vi "SDO_TRAJECTORY_EXECUTE_ABS.vi"(6 "EnableClosedLoop":bool=TRUE, 8 "Init":bool, 11 "End Pose ENG":T1={"TRANSLATION"={"X"=0.0, "Y"=0.0}, "ROTATION"={"VALUE"=0.0, "COS"=1.0, "SIN"=0.0}} {"ROTATION"."SIN" format="%13.4f"; "ROTATION"."COS" format="%13.4f"; "ROTATION"."VALUE" format="%13.4f"; "TRANSLATION"."Y" format="%14.3f"; "TRANSLATION"."X" format="%14.3f"}) -> (0 "AtReference":bool, 3 "Chassis Velocity Target":T4 {"vOmega" format="%10.3f"; "vY" format="%10.3f"; "vX" format="%10.3f"})   [LabVIEW 2019]
uses:
  <vilib>/Rock Robotics/WPI/ThirdParty/JAS_Junk/TrajLib/TypeDef/CHASSIS_SPEEDS.ctl
  <vilib>/Rock Robotics/WPI/ThirdParty/JAS_Junk/TrajLib/TypeDef/POSE2D.ctl
  <vilib>/Rock Robotics/WPI/ThirdParty/JAS_Junk/TrajLib/TypeDef/TRANSLATION2D.ctl
  <vilib>/Rock Robotics/WPI/ThirdParty/JAS_Junk/TrajLib/TypeDef/ROTATION2D.ctl
  <vilib>/Rock Robotics/WPI/ThirdParty/JAS_Junk/TrajLib/VI/Util_GetTime_U32.vi
  <vilib>/Rock Robotics/WPI/ThirdParty/JAS_Junk/TrajLib/ProfiledPIDController_NewPeriod.vi
  <vilib>/Rock Robotics/WPI/ThirdParty/JAS_Junk/TrajLib/ProfiledPIDController_SetIntegratorRange.vi
  <vilib>/Rock Robotics/WPI/ThirdParty/JAS_Junk/TrajLib/ProfiledPIDController_DisableContInput.vi
  <vilib>/Rock Robotics/WPI/ThirdParty/JAS_Junk/TrajLib/ProfiledPIDController_EnableContInput.vi
  <vilib>/Rock Robotics/WPI/ThirdParty/JAS_Junk/TrajLib/TrapProfConstraint_New.vi
  <vilib>/Rock Robotics/WPI/ThirdParty/JAS_Junk/TrajLib/HolDrvCtrl_New.vi
  <vilib>/Rock Robotics/WPI/ThirdParty/JAS_Junk/TrajLib/HolDrvCtrl_PackPID.vi
  <vilib>/Rock Robotics/WPI/ThirdParty/JAS_Junk/TrajLib/HolDrvCtrl_SetTolerance.vi
  <vilib>/Rock Robotics/WPI/ThirdParty/JAS_Junk/TrajLib/HolDrvCtrl_SetEnabled.vi
  <vilib>/Rock Robotics/WPI/ThirdParty/JAS_Junk/TrajLib/HolDrvCtrl_Calculate_Trajectory.vi
  <vilib>/Rock Robotics/WPI/ThirdParty/JAS_Junk/TrajLib/HolDrvCtrl_AtReference.vi
  <vilib>/Rock Robotics/WPI/ThirdParty/JAS_Junk/TrajLib/TrapProfState_New.vi
  <vilib>/Rock Robotics/WPI/ThirdParty/JAS_Junk/TrajLib/PIDController_NewPeriod.vi
  <vilib>/Rock Robotics/SystemInterfaces/NetworkCommunication/NetComm_UsageReport_report.vi
  <vilib>/Rock Robotics/WPI/ThirdParty/JAS_Junk/TrajLib/PIDController_SetIntegratorRange.vi
  <vilib>/Rock Robotics/WPI/ThirdParty/JAS_Junk/TrajLib/PIDController_DisableContinousInput.vi
  <vilib>/Rock Robotics/WPI/ThirdParty/JAS_Junk/TrajLib/PIDController_EnableContinousInput.vi
  <vilib>/Rock Robotics/WPI/ThirdParty/JAS_Junk/TrajLib/Conv_Deg_Radians.vi
  <vilib>/Rock Robotics/WPI/ThirdParty/JAS_Junk/TrajLib/PIDController_Reset.vi
  <vilib>/Rock Robotics/WPI/ThirdParty/JAS_Junk/TrajLib/HolDrvCtrl_Calculate.vi
  <vilib>/Rock Robotics/WPI/ThirdParty/JAS_Junk/TrajLib/Rotation2d_GetRadians.vi
  <vilib>/Rock Robotics/WPI/ThirdParty/JAS_Junk/TrajLib/Rotation2d_GetAngleCosSin.vi
  <vilib>/Rock Robotics/WPI/ThirdParty/JAS_Junk/TrajLib/Pose2d_RelativeTo.vi
  <vilib>/Rock Robotics/WPI/ThirdParty/JAS_Junk/TrajLib/Pose2d_getRotation.vi
  <vilib>/Rock Robotics/WPI/ThirdParty/JAS_Junk/TrajLib/Rotation2d_Minus.vi
  <vilib>/Rock Robotics/WPI/ThirdParty/JAS_Junk/TrajLib/ProfiledPIDController_Calculate_Meas_Goal.vi
  <vilib>/Rock Robotics/WPI/ThirdParty/JAS_Junk/TrajLib/ChassisSpeeds_FromFieldRelativeSpeeds.vi
  <vilib>/Rock Robotics/WPI/ThirdParty/JAS_Junk/TrajLib/PIDController_Calculate_SP_PV.vi
  <vilib>/Rock Robotics/WPI/ThirdParty/JAS_Junk/TrajLib/ProfiledPIDController_Reset_PosOnly.vi
  <vilib>/Rock Robotics/WPI/ThirdParty/JAS_Junk/TrajLib/Transform2d_Create_PosePose.vi
  <vilib>/Rock Robotics/WPI/ThirdParty/JAS_Junk/TrajLib/Pose2d_New_TRRO.vi
  <vilib>/Rock Robotics/WPI/ThirdParty/JAS_Junk/TrajLib/Rotation2d_UnaryMinus.vi
  <vilib>/Rock Robotics/WPI/ThirdParty/JAS_Junk/TrajLib/Rotation2d_RotateBy.vi
  <vilib>/Rock Robotics/WPI/ThirdParty/JAS_Junk/TrajLib/ProfiledPIDController_SetGoal_PosOnly.vi
  <vilib>/Rock Robotics/WPI/ThirdParty/JAS_Junk/TrajLib/ProfiledPIDController_Calculate_Meas.vi
  <vilib>/Rock Robotics/WPI/ThirdParty/JAS_Junk/TrajLib/Rotation2d_GetCos.vi
  <vilib>/Rock Robotics/WPI/ThirdParty/JAS_Junk/TrajLib/Rotation2d_GetSin.vi
  <vilib>/Rock Robotics/WPI/ThirdParty/JAS_Junk/TrajLib/PIDController_SetSetpoint.vi
  <vilib>/Rock Robotics/WPI/ThirdParty/JAS_Junk/TrajLib/PIDController_Calculate_PV.vi
  <vilib>/Rock Robotics/WPI/ThirdParty/JAS_Junk/TrajLib/ProfiledPIDController_Reset.vi
  <vilib>/Rock Robotics/WPI/ThirdParty/JAS_Junk/TrajLib/Translation2d_RotateBy.vi
  <vilib>/Rock Robotics/WPI/ThirdParty/JAS_Junk/TrajLib/Translation2d_Minus.vi
  <vilib>/Rock Robotics/WPI/ThirdParty/JAS_Junk/TrajLib/Rotation2d_CreateAngle.vi
  <vilib>/Rock Robotics/WPI/ThirdParty/JAS_Junk/TrajLib/Rotation2d_CreateXY.vi
  <vilib>/Rock Robotics/WPI/ThirdParty/JAS_Junk/TrajLib/ProfiledPIDController_SetGoal.vi
  <vilib>/Rock Robotics/WPI/ThirdParty/JAS_Junk/TrajLib/TrapProfile_New.vi
  <vilib>/Rock Robotics/WPI/ThirdParty/JAS_Junk/TrajLib/ProfiledPIDController_GetPeriod.vi
  <vilib>/Rock Robotics/WPI/ThirdParty/JAS_Junk/TrajLib/TrapProfile_Calculate.vi
  <vilib>/Rock Robotics/WPI/ThirdParty/JAS_Junk/TrajLib/ControllerUtil_GetModulusError.vi
  <vilib>/Rock Robotics/WPI/ThirdParty/JAS_Junk/TrajLib/Translation2d_Create.vi
  <vilib>/Rock Robotics/WPI/ThirdParty/JAS_Junk/TrajLib/Util_CalcDist.vi
  <vilib>/Rock Robotics/WPI/ThirdParty/JAS_Junk/TrajLib/TrapProfile_ShouldFlipAcceleration.vi
  <vilib>/Rock Robotics/WPI/ThirdParty/JAS_Junk/TrajLib/TrapProfile_Direct.vi
  <vilib>/Rock Robotics/WPI/ThirdParty/JAS_Junk/TrajLib/PIDController_GetPeriod.vi
  <vilib>/Rock Robotics/WPI/ThirdParty/JAS_Junk/TrajLib/VI/Util_GetTime_U64.vi
  SDO_TRAJECTORY_GLOBALS.vi
  <vilib>/Rock Robotics/WPI/ThirdParty/JAS_Junk/TrajLib/Globals/Util_LibraryGlobals.vi
  Swerve_Drive_System/SDO_DRIVE_GLOBALS.vi
  <vilib>/Rock Robotics/WPI/ThirdParty/JAS_Junk/TrajLib/Trajectory_Library.lvlib
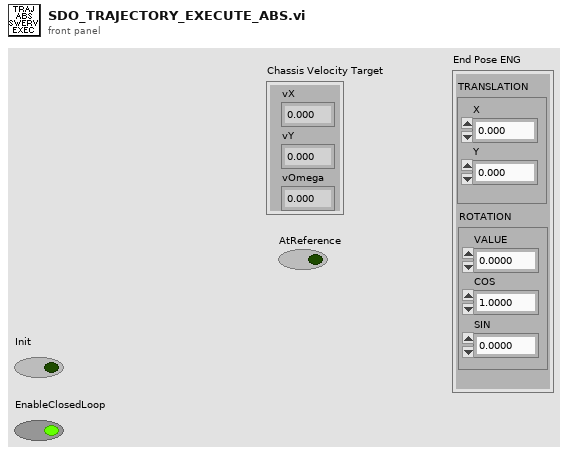
[diagram p1: front panel]
types:
  T1 = typedef "Trajectory_Library.lvlib/POSE2D.ctl" = cluster{"TRANSLATION":T2, "ROTATION":T3}
  T2 = typedef "Trajectory_Library.lvlib/TRANSLATION2D.ctl" = cluster{"X":dbl, "Y":dbl}
  T3 = typedef "Trajectory_Library.lvlib/ROTATION2D.ctl" = cluster{"VALUE":dbl, "COS":dbl, "SIN":dbl}
  T4 = typedef "Trajectory_Library.lvlib/CHASSIS_SPEEDS.ctl" = cluster{"vX":dbl, "vY":dbl, "vOmega":dbl}
  T5 = typedef "Trajectory_Library.lvlib/SWERVE_DRIVE_KINEMATICS.ctl" = cluster{"NumModules":i32, "InverseKinematics":T6, "ForwardKinematics":T6, "Modules":T2[], "PrevCoR":T2, "SavedModuleStates":T7[]}
  T6 = typedef "NI_Matrix.lvlib/RealMatrix.ctl" = dbl[][]
  T7 = typedef "Trajectory_Library.lvlib/SWERVE_DRIVE_MODULE_STATE.ctl" = cluster{"Speed":dbl, "Angle":T3}
  T8 = typedef "Trajectory_Library.lvlib/TRAJECTORY.ctl" = cluster{"TotalTImeSecs":dbl, "States":T9[]}
  T9 = typedef "Trajectory_Library.lvlib/TRAJ_STATE.ctl" = cluster{"TimeSeconds":dbl, "Velocity":dbl, "Acceleration":dbl, "POSE":T1, "Curvature":dbl}
  T10 = typedef "Trajectory_Library.lvlib/PID_TUNING.ctl" = cluster{"Kp":dbl, "Ki":dbl, "Kd":dbl, "MaximumIntegral":dbl, "MinimumIntegral":dbl}
  T11 = typedef "Trajectory_Library.lvlib/PROFILED_PID_CONTROLLER.ctl" = cluster{"Controller":T12, "Goal":T13, "Setpoint":T13, "Constraint":T14}
  T12 = typedef "Trajectory_Library.lvlib/PID_CONTROLLER.ctl" = cluster{"Kp":dbl, "Ki":dbl, "Kd":dbl, "Period":dbl, "Max_Integral":dbl, "Min_Integral":dbl, "Max_Input":dbl, "Min_Input":dbl, "Continuous":bool, "PositionError":dbl, "VelocityError":dbl, "PrevError":dbl, "TotalError":dbl, "PositionTolerance":dbl, "VelocityTolerance":dbl, "SetPoint":dbl, "Kf":dbl, "Prev_Deriv":dbl, "Prev_Deriv 2":dbl, "DerivativeFilter":bool, "Min_Output":dbl, "Max_Output":dbl, "Prev_F_P":dbl, "Prev_F_P_2":dbl, "AntiWindupActive":bool, "Measurement":dbl}
  T13 = typedef "Trajectory_Library.lvlib/TRAPEZOID_PROFILE_STATE.ctl" = cluster{"Position":dbl, "Velocity":dbl}
  T14 = typedef "Trajectory_Library.lvlib/TRAPEZOID_PROFILE_CONSTRAINT.ctl" = cluster{"MaxVelocity":dbl, "MaxAcceleration":dbl}
  T15 = typedef "Trajectory_Library.lvlib/HOLONOMIC_PACK_TUNING.ctl" = cluster{"X PID Tuning":T10, "Y PID Tuning":T10, "thetaProfiledPID_CTRL":T11}
  T16 = typedef "Trajectory_Library.lvlib/HOLONOMIC_DRV_CTRL.ctl" = cluster{"poseTolerance":T1, "poseError":T1, "Enabled":bool, "PID_xCtrl":T12, "PID_yCtrl":T12, "PROF_PID_thetaCtrl":T11, "RotationError":T3, "FirstRun":bool}
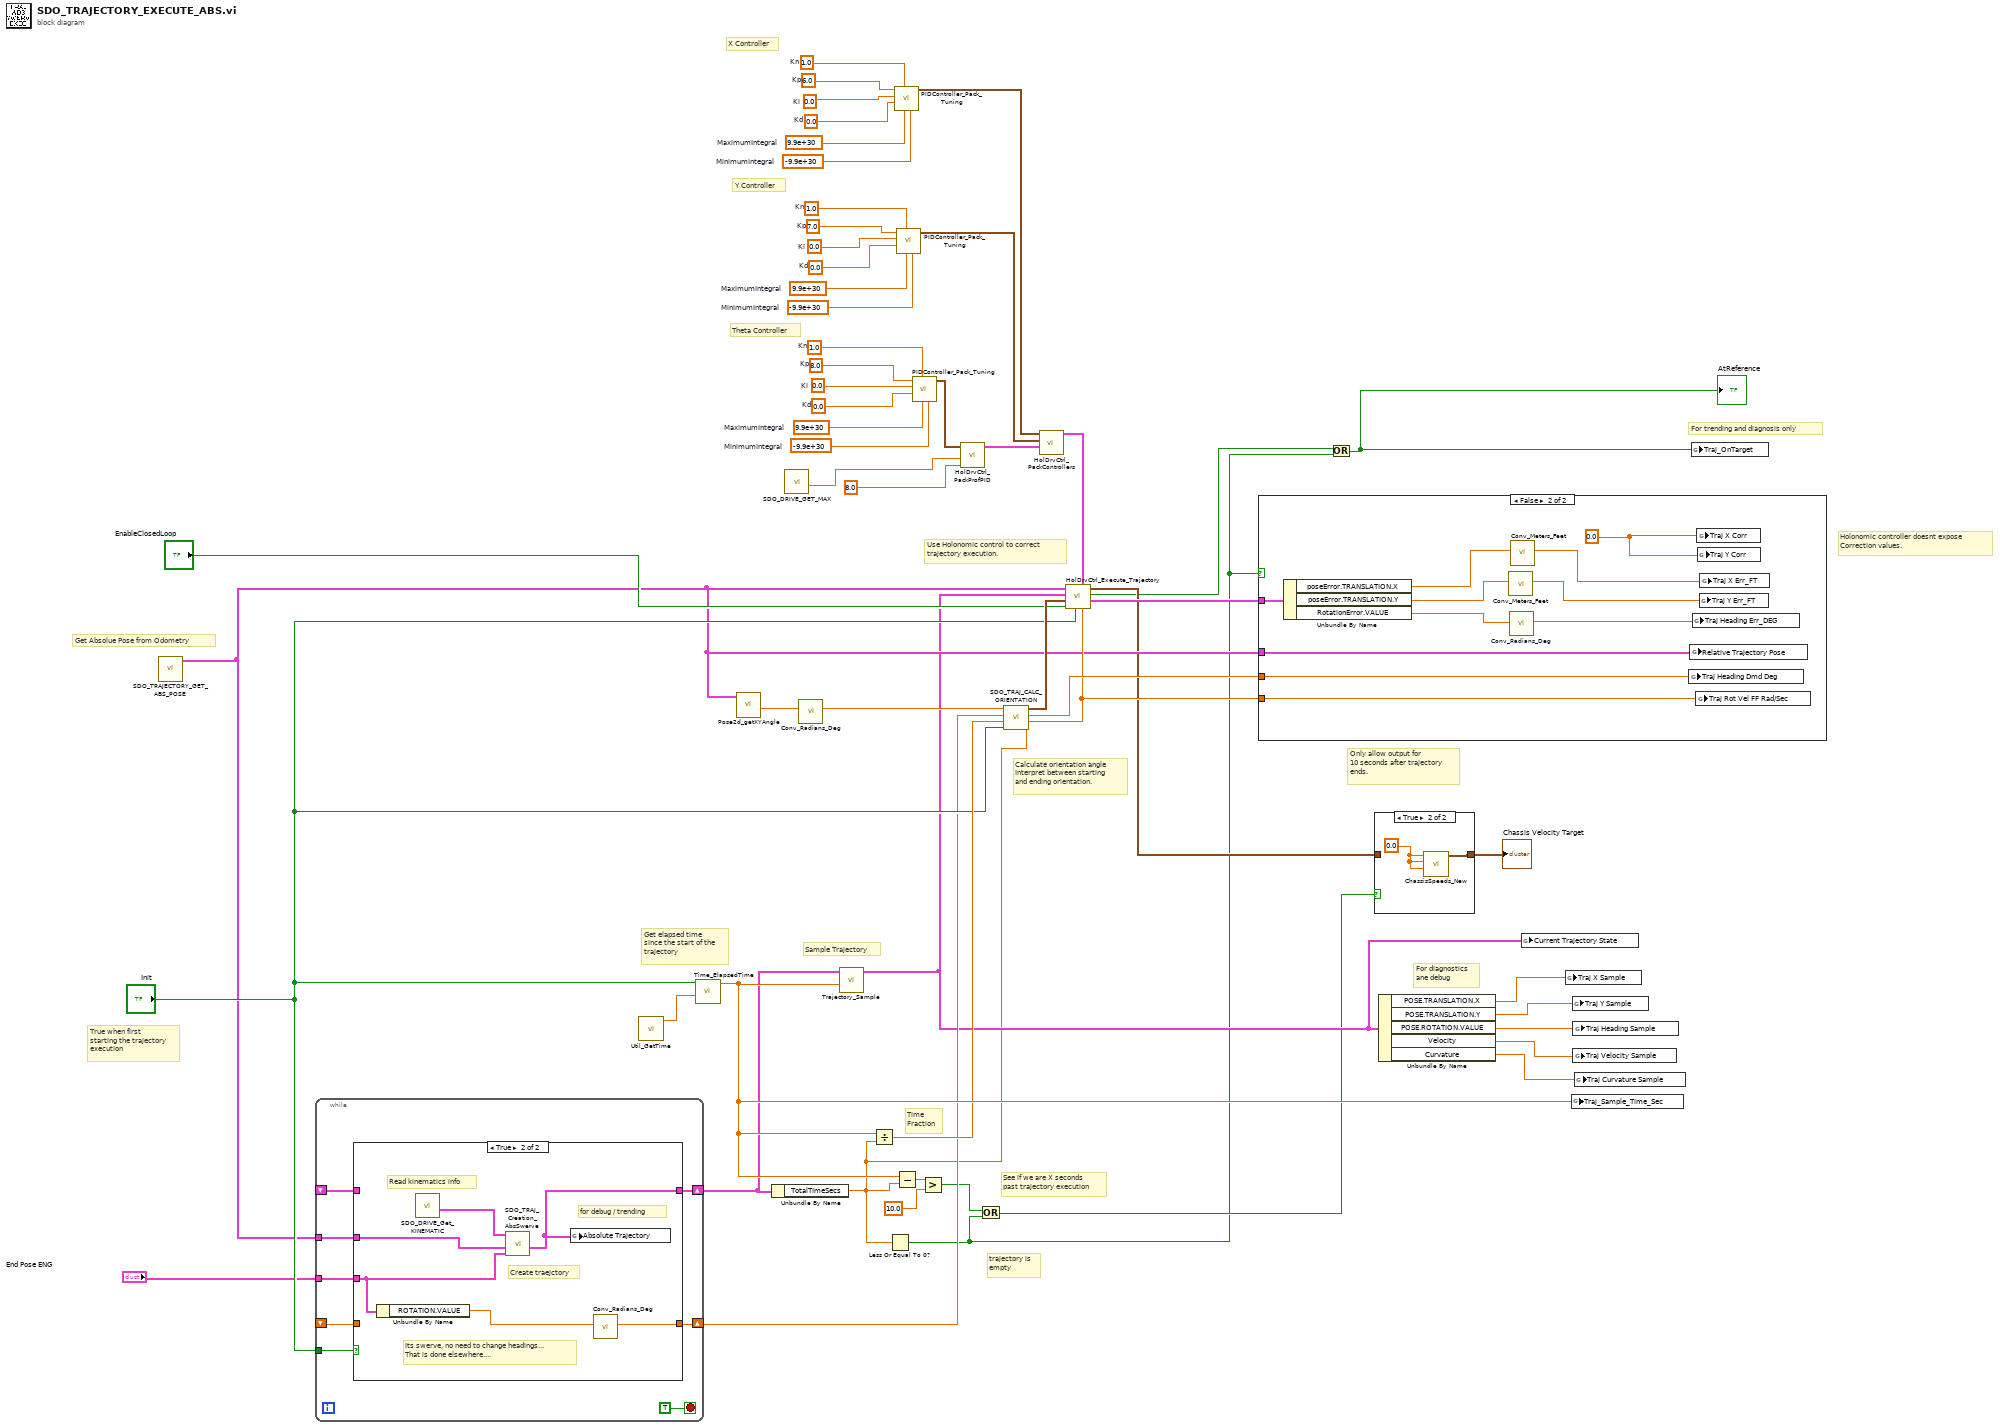
[diagram p0: block diagram]
diagram:
  w25 = 1.0  # Kn
  w28 = 8.0  # Kp
  w37 = 0.0  # Ki
  w38 = 0.0  # Kd
  w39 = 9.9e+30  # MaximumIntegral
  w40 = -9.9e+30  # MinimumIntegral
  w23 = 1.0  # Kn
  w26 = 6.0  # Kp
  w29 = 0.0  # Ki
  w30 = 0.0  # Kd
  w31 = 9.9e+30  # MaximumIntegral
  w32 = -9.9e+30  # MinimumIntegral
  w24 = 1.0  # Kn
  w27 = 7.0  # Kp
  w33 = 0.0  # Ki
  w34 = 0.0  # Kd
  w35 = 9.9e+30  # MaximumIntegral
  w36 = -9.9e+30  # MinimumIntegral
  # "trajectory is \nempty"
  # "Theta Controller"
  # "Y Controller"
  # "X Controller"
  # "Time\nFraction"
  # "Calculate orientation angle\nInterpret between starting\nand ending orientation."
  # "True when first\nstarting the trajectory\nexecution"
  # "Get elapsed time\nsince the start of the\ntrajectory"
  # "Holonomic controller doesnt expose\nCorrection values."
  # "Use Holonomic control to correct\ntrajectory execution."
  # "For trending and diagnosis only"
  # "For diagnostics\nane debug"
  # "Get Absolue Pose from Odometry"
  # "Sample Trajectory"
  # "See if we are X seconds \npast trajectory execution"
  # "Only allow output for\n10 seconds after trajectory\nends."
  n1 = call "SDO_TRAJECTORY_GET_ABS_POSE.vi"() -> ("Absolute Odometry Pose"=w13:T1)  [unwired: 11 in]
  n2 = while {
    tunnel: "Init" -> [w63]
    tunnel: w13 -> [w62]
    shift-right: [w61] -> w14
    shift-left: _ -> [w60]
    shift-right: [w59] -> w10
    shift-left: _ -> [w58]
    tunnel: "End Pose ENG" -> [w57]
    stop <- TRUE stop-if-true
    n3 = case shown="True" w63 {
      tunnel: w62 -> [_ w68]
      tunnel: [w66 w69] -> w61
      tunnel: w60 -> [w66 _]
      tunnel: [w65 w71] -> w59
      tunnel: w58 -> [w65 _]
      tunnel: w57 -> [_ w72]
      frame False {
      }
      frame True {
        # "for debug / trending"
        # "Read kinematics info"
        # "Its swerve, no need to change headings...\nThat is done elsewhere...."
        # "Create traejctory"
        n4 = Unbundle By Name(w72) -> ("ROTATION.VALUE"=w70:dbl)
        n5 = call "SDO_DRIVE_Get_KINEMATIC.vi"() -> ("out SWERVE_DRIVE_KINEMATICS"=w67:T5)  [unwired: 11 in]
        n6 = call "SDO_TRAJ_Creation_AbsSwerve.vi"("End Pose  ENG"=w72, "Current Pose SI"=w68, "SWERVE_DRIVE_KINEMATICS"=w67) -> ("Absolute Trajectory"=w69:T8)  [unwired: 6 in, 2 out]
        n7 = global write "SDO_TRAJECTORY_GLOBALS.vi" "Absolute Trajectory"(w69) -> ()
        n8 = call <vilib>:"Conv_Radians_Deg.vi"("Radians"=w70) -> ("Degrees"=w71:dbl)  [unwired: 10 in]
      }
    }
  }
  n9 = call <vilib>:"Util_GetTime.vi"() -> ("FPGA_Time_Seconds"=w53:dbl)  [unwired: 9 in, 2 out]
  n10 = call <vilib>:"Time_ElapsedTime.vi"("PassthroughTime_SEC"=w53, "Reset"="Init") -> ("Elapsed Time Sec"=w46:dbl)  [unwired: 9 in]
  n11 = call <vilib>:"Pose2d_getXYAngle.vi"("in POSE"=w13) -> ("Angle"=w12:dbl)  [unwired: 8 in, 2 out]
  n12 = Unbundle By Name(w14) -> ("TotalTImeSecs"=w6:dbl)
  n13 = call "SDO_DRIVE_GET_MAX.vi"() -> ("Max Rotational Vel (Rad/Sec)"=w17:dbl)  [unwired: 10 in, 1 out]
  n14 = call <vilib>:"Conv_Radians_Deg.vi"("Radians"=w12) -> ("Degrees"=w11:dbl)  [unwired: 10 in]
  n15 = call <vilib>:"Trajectory_Sample.vi"("Time"=w46, "InputTRAJECTORY"=w14) -> ("OutputTRAJ_STATE"=w9:T9)  [unwired: 9 in]
  n16 = Divide(x=w46, y=w6) -> (x/y=w45:dbl)
  n17 = Less Or Equal To 0?(x=w6) -> (x <= 0?=w1:bool)
  n18 = call <vilib>:"PIDController_Pack_Tuning.vi"("MinimumIntegral"=w32, "MaximumIntegral"=w31, "Kn"=w23, "Kd"=w30, "Ki"=w29, "Kp"=w26) -> ("PID Tuning"=w41:T10)  [unwired: 5 in]
  n19 = Subtract(x=w46, y=w6) -> (x-y=w56:dbl)
  n20 = call <vilib>:"PIDController_Pack_Tuning.vi"("MinimumIntegral"=w36, "MaximumIntegral"=w35, "Kn"=w24, "Kd"=w34, "Ki"=w33, "Kp"=w27) -> ("PID Tuning"=w42:T10)  [unwired: 5 in]
  n21 = call <vilib>:"PIDController_Pack_Tuning.vi"("MinimumIntegral"=w40, "MaximumIntegral"=w39, "Kn"=w25, "Kd"=w38, "Ki"=w37, "Kp"=w28) -> ("PID Tuning"=w22:T10)  [unwired: 5 in]
  n22 = Greater?(x=w56, y=10.0) -> (0:w5:bool)
  n23 = call <vilib>:"HolDrvCtrl_PackProfPID.vi"("Max Accel"=8.0, "Max Speed"=w17, "Theta PID Tuning"=w22) -> ("Theta PID CONTROLLER"=w43:T11)  [unwired: 8 in]
  n24 = Or(x=w5, y=w1) -> (x .or. y?=w4:bool)
  n25 = call "SDO_TRAJ_CALC_ORIENTATION.vi"("Total Trajectory Time"=w6, "Init"="Init", "Time Fraction"=w45, "End Orientation Demand DEG"=w10, "Starting Orientation  DEG"=w11) -> ("Rotational Velocity Rad Per Sec"=w19:dbl, 2:"Orientation Demand Deg"=w47:dbl, 3:"Orientation Demand Deg"=w21:T3)  [unwired: 4 in]
  n26 = call <vilib>:"HolDrvCtrl_PackControllers.vi"("thetaProfiledPID_CTRL"=w43, "Y PID Tuning"=w42, "X PID Tuning"=w41) -> ("HOLONOMIC_CTRL_PACK_TUNING"=w44:T15)  [unwired: 8 in]
  n27 = call <vilib>:"HolDrvCtrl_Execute_Trajectory.vi"("Rotational Velocity Feedforward \nRad/Sec"=w19, "HOLONOMIC_CTRL_PACK_TUNING"=w44, "Reset"="Init", "Enable"="EnableClosedLoop", "angleRef"=w21, "desiredTrajState"=w9, "currentPose"=w13) -> ("outHOLONOMIC_DRV_CTRL"=w20:T16, "AtReference"=w3:bool, "calcChassisSpeed"=w7:T4)  [unwired: 2 in]
  n28 = case shown="False" w1 {
    tunnel: w47 -> [_ w82]
    tunnel: w20 -> [_ w76]
    tunnel: w19 -> [_ w75]
    tunnel: w13 -> [_ w73]
    frame True {
    }
    frame False {
      w83 = 0.0 ("Y Corr")
      n29 = Unbundle By Name(w76) -> ("poseError.TRANSLATION.X"=w80:dbl, "poseError.TRANSLATION.Y"=w79:dbl, "RotationError.VALUE"=w74:dbl)
      n30 = call <vilib>:"Conv_Meters_Feet.vi"("Meters"=w79) -> ("Feet"=w78:dbl)  [unwired: 10 in]
      n31 = call <vilib>:"Conv_Radians_Deg.vi"("Radians"=w74) -> ("Degrees"=w81:dbl)  [unwired: 10 in]
      n32 = call <vilib>:"Conv_Meters_Feet.vi"("Meters"=w80) -> ("Feet"=w77:dbl)  [unwired: 10 in]
      n33 = global write "SDO_TRAJECTORY_GLOBALS.vi" "Traj Heading Dmd Deg"(w82) -> ()
      n34 = global write "SDO_TRAJECTORY_GLOBALS.vi" "Relative Trajectory Pose"(w73) -> ()
      n35 = global write "SDO_TRAJECTORY_GLOBALS.vi" "Traj Heading Err_DEG"(w81) -> ()
      n36 = global write "SDO_TRAJECTORY_GLOBALS.vi" "Traj Rot Vel FF Rad/Sec"(w75) -> ()
      n37 = global write "SDO_TRAJECTORY_GLOBALS.vi" "Traj X Corr"(w83) -> ()
      n38 = global write "SDO_TRAJECTORY_GLOBALS.vi" "Traj Y Corr"(w83) -> ()
      n39 = global write "SDO_TRAJECTORY_GLOBALS.vi" "Traj Y Err_FT"(w78) -> ()
      n40 = global write "SDO_TRAJECTORY_GLOBALS.vi" "Traj X Err_FT"(w77) -> ()
    }
  }
  n41 = Or(x=w3, y=w1) -> (x .or. y?=w2:bool)
  "AtReference" <- w2
  n42 = case shown="True" w4 {
    tunnel: w7 -> [w84 _]
    tunnel: [w84 w85] -> w54
    frame False {
    }
    frame True {
      w86 = 0.0 ("vX")
      n43 = call <vilib>:"ChassisSpeeds_New.vi"("vAngular"=w86, "vY"=w86, "vX"=w86) -> ("CHASSIS"=w85:T4)  [unwired: 8 in]
    }
  }
  "Chassis Velocity Target" <- w54
  n44 = Unbundle By Name(w9) -> ("POSE.TRANSLATION.X"=w52:dbl, "POSE.TRANSLATION.Y"=w51:dbl, "POSE.ROTATION.VALUE"=w50:dbl, "Velocity"=w49:dbl, "Curvature"=w48:dbl)
  n45 = global write "SDO_TRAJECTORY_GLOBALS.vi" "Current Trajectory State"(w9) -> ()
  n46 = global write "SDO_TRAJECTORY_GLOBALS.vi" "Traj X Sample"(w52) -> ()
  n47 = global write "SDO_TRAJECTORY_GLOBALS.vi" "Traj_Sample_Time_Sec"(w46) -> ()
  n48 = global write "SDO_TRAJECTORY_GLOBALS.vi" "Traj Y Sample"(w51) -> ()
  n49 = global write "SDO_TRAJECTORY_GLOBALS.vi" "Traj Heading Sample"(w50) -> ()
  n50 = global write "SDO_TRAJECTORY_GLOBALS.vi" "Traj Velocity Sample"(w49) -> ()
  n51 = global write "SDO_TRAJECTORY_GLOBALS.vi" "Traj Curvature Sample"(w48) -> ()
  n52 = global write "SDO_TRAJECTORY_GLOBALS.vi" "Traj_OnTarget"(w2) -> ()
